vi "tcsOfc_getEvent_noEnoughZernikeTerm.vi"(8 "error in (no error)":errorcluster, 11 "logevent_noEnoughZernikeTerm_Ctl":T1) -> (0 "error out":errorcluster, 2 "function return":i32, 3 "logevent_noEnoughZernikeTerm_Ctl out":T1)   [LabVIEW 2016, in "SALLV_tcsOfc.lvlib"]
doc: "int tcsOfc_shm_getEvent_noEnoughZernikeTermLV(tcsOfc_logevent_noEnoughZernikeTermLV *logevent_noEnoughZernikeTerm_Ctl );"
uses:
  SALLV_tcsOfc.lvlib
  DataTypes/logevent_noEnoughZernikeTerm.ctl
  SALLV_tcsOfc.so
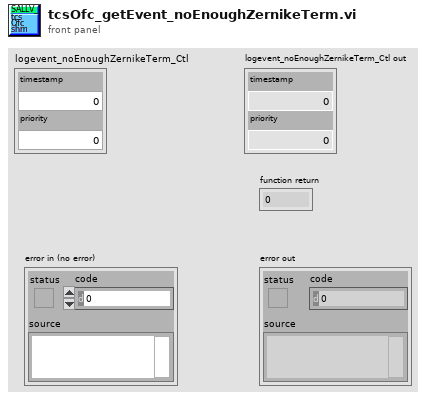
[diagram p1: front panel]
types:
  T1 = typedef "SALLV_tcsOfc.lvlib/logevent_noEnoughZernikeTerm.ctl" = cluster{"timestamp":dbl, "priority":i32}
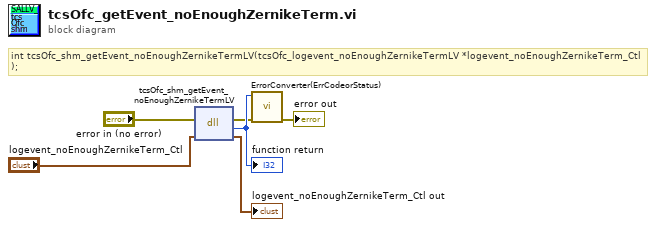
[diagram p0: block diagram]
diagram:
  # "int tcsOfc_shm_getEvent_noEnoughZernikeTermLV(tcsOfc_logevent_noEnoughZernikeTermLV *logevent_noEnoughZernikeTerm_Ctl );"
  n1 = dll-call lib="home/andres/Desktop/SAL_tcsOfc/SALLV_tcsOfc.*" fn="tcsOfc_shm_getEvent_noEnoughZernikeTermLV"(error in="error in (no error)", "logevent_noEnoughZernikeTerm_Ctl"="logevent_noEnoughZernikeTerm_Ctl") -> (error out=w2:errorcluster, w6:i32, "logevent_noEnoughZernikeTerm_Ctl"=→"logevent_noEnoughZernikeTerm_Ctl out":T1)  [unwired: 2 in, 1 out]
  "function return" <- w6
  n2 = call "ErrorConverter(ErrCodeorStatus).vi"("error in (no error)"=w2, "error code"=w6) -> ("error out"=→"error out":errorcluster)  [unwired: 9 in]
